vi "FA_AgentConfig_Close.vi"(8 "Error In":errorcluster, 11 "FA_AgentConfig_Refnum 2":T1) -> (0 "Error Out":errorcluster)   [LabVIEW 2013, in "FA_AgentConfig.lvlib"]
uses:
  FA_AgentConfig.lvlib
  FA_AgentConfig_Refnum.ctl
  <vilib>/Utility/config.llb/Config Data RefNum.ctl
  <vilib>/Utility/config.llb/NI_LVConfig.lvlib
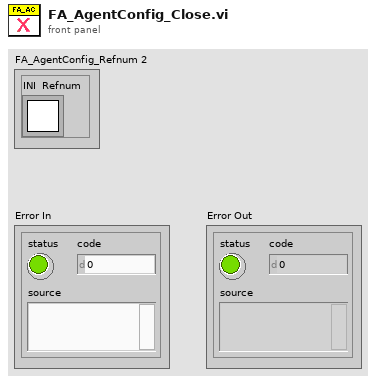
[diagram p1: front panel]
types:
  T1 = typedef "FA_AgentConfig.lvlib/FA_AgentConfig_Refnum.ctl" = cluster{"INI  Refnum":T2}
  T2 = typedef "NI_LVConfig.lvlib/Config Data RefNum.ctl" = refnum<k1>
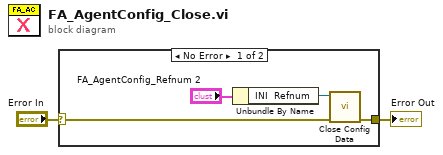
[diagram p0: block diagram]
diagram:
  n1 = case shown="No Error" "Error In" {
    selector: "Error In" -> [w4 w7]
    tunnel: [w3 w7] -> w1
    frame No Error {
      n2 = Unbundle By Name("FA_AgentConfig_Refnum 2") -> ("INI  Refnum"=w6:T2)
      n3 = call <vilib>:"Close Config Data.vi"("error in (no error)"=w4, "refnum"=w6) -> ("error out"=w3:errorcluster)  [unwired: 8 in, 1 out]
    }
    frame Error {
    }
  }
  "Error Out" <- w1
